vi "Get_Motor_Position.vi"(4 "Echo Mode (2)":i32=2, 6 "additional witing time (0)":u32, 7 "Motor In":u16(ring) items=["none", "1", "2", "3", "4", "all"], 8 "error in (no error)":errorcluster, 10 "Output Unit":T1=enum."Angle [TMC]", 11 "VISA resource name":refnum<visa-resource-name>) -> (0 "error out":errorcluster={"status"=FALSE, "code"=1073676294, "source"="VISA Read in write_read.vi"}, 1 "Position (Steps)":i32, 2 "Position":dbl, 3 "VISA ressource out":refnum<visa-resource-name>)   [LabVIEW 2018]
uses:
  ConversionAndInformation/Unit_Control.ctl
  MCode_LV_86/Set Parameter.ctl
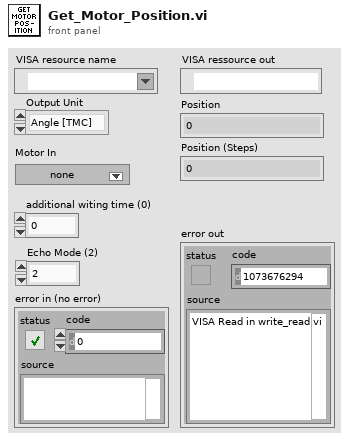
[diagram p1: front panel]
types:
  T1 = typedef "Unit_Control.ctl" = enum16{"Angle (Degrees)", "Rad", "Angle [TMC]", "Microsteps [TMC]", "Inches", "Nanometer", "Meter", "Centimeter", "Millimeter", "Micron"}
  T2 = typedef "Set Parameter.ctl" = enum16{"Acceleration (A)", "Baud Rate (BD)", "Counter 1 (C1)", "Counter 2 (C2)", "Control C Software Reset (CE)", "Check Sum Enable (CK)", "Clock Mode (CM)", "Clock Mode Ratio (CR)", "Clock Mode Out Step Width (CW)", "Deceleration (D)", "Digital Filtering, Input 1 (D1)", "Digital Filtering, Input 2 (D2)", "Digital Filtering, Input 3 (D3)", "Digital Filtering, Input 4 (D4)", "Digital Filtering, Input 5 (D5)", "Digital Filtering, Input 9 (D9)", "Digital Filtering, Input 10 (D10)", "Digital Filtering, Input 11 (D11)", "Digital Filtering, Input 12 (D12)", "Deadband (DB)", "Decrement Variable (DC)", "Enable/Disable Drive (DE)", "Device Name (DN)", "End Program Execution (E)", "Encoder Function Enable (EE)", "Error Flag (EF)", "Encoder Lines (EL)", "Echo Mode (EM)", "Error Value (ER)", "Escape (ES)", "Execute Program at Address (EX)", "Firmware Version (VR)", "Hold (H)", "Hold Current (HC)", "Hold Current Delay Time (HI)", "Home to Encoder Index (HM)", "Home to Home Switch (HT)", "Increment Variable (IC)", "Initialize Parameters to NVM (IP)", "Input into Variable (IV)", "Jog Enable (JE)", "Limit Stop Mode (LM)", "Move Absolute (MA)", "Move Relative (MR)", "MicroStepping Select (MS)", "Motor Settling Delay Time (MT)", "Moving [Flag] (MV)", "Output 1 (O1)", "Output 2 (O2)", "Output 3 (O3)", "Output 4 (O4)", "Output 9 (O9)", "Output 10 (O10)", "Output 11 (O11)", "Output 12 (O12)", "Output High Byte (9-12) (OH)", "Output Low Byte (1-4) (OL)", "Output Total (1-4 and 9-12) (OT)", "Position (P)", "Position Maintenance (PM)", "Party Mode (PY)", "Register 1 (R1)", "Register 2 (R2)", "Register 3 (R3)", "Register 4 (R4)", "Reset Error(\\03)", "Run Current (RC)", "Stall Factor (SF)", "Slew (SL)", "Stall Mode Set (SM)", "Upgrade Firmware (UG)", "Velocity Initial (VI)", "Velocity Maximum (VM)", "Current1 (I1)", "Current2 (I2)", "Current3 (I3)", "Current4 (I4)", "Current5 (I5)", "Current6 (I6)", "Save (S)"}
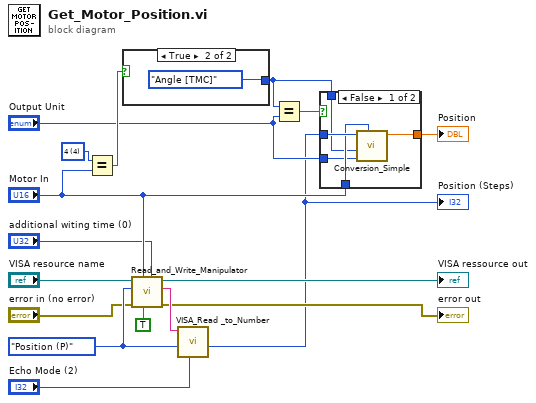
[diagram p0: block diagram]
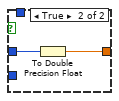
[diagram p2: hidden frame]
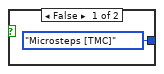
[diagram p3: hidden frame]
diagram:
  w9 = u16 4 items=["none", "1", "2", "3", "4", "all"] ("Motor")
  w15 = Set_Parameter."Position (P)" ("Command")
  n1 = Equal?(x=w9, y="Motor In") -> (x = y?=w7:bool)
  n2 = case shown="True" w7 {
    tunnel: [Unit_Control."Microsteps [TMC]" ("Input Unit") Unit_Control."Angle [TMC]" ("Input Unit")] -> w4
    frame False {
    }
    frame True {
    }
  }
  n3 = call "Read_and_Write_Manipulator.vi"("additional waiting time (0)"="additional witing time (0)", "Print?"=TRUE, "Motor"="Motor In", "error in (no error)"="error in (no error)", "Command"=w15, "VISA resource name"="VISA resource name") -> ("error out"=→"error out":errorcluster, "Answer"=w16:string, "VISA ressource out"=→"VISA ressource out":refnum<visa-resource-name>)  [unwired: 1 in, 2 out]
  n4 = call "VISA_Read _to_Number.vi"("Echo Mode"="Echo Mode (2)", "Command"=w15, "Answer Buffer"=w16) -> ("number (I32)"=w3:i32)  [unwired: 7 in, 1 out]
  "Position (Steps)" <- w3
  n5 = Equal?(x=w4, y="Output Unit") -> (x = y?=w6:bool)
  n6 = case shown="False" w6 {
    tunnel: w3 -> [w24 w26]
    tunnel: [w23 w25] -> w14
    tunnel: "Motor In" -> [w22 _]
    tunnel: w4 -> [w21 _]
    tunnel: "Output Unit" -> [w20 _]
    frame False {
      n7 = call "Conversion_Simple.vi"("Motor"=w22, "Output Unit"=w20, "Input Unit"=w21, "Input"=w24) -> ("Output"=w23:dbl)  [unwired: 6 in, 1 out]
    }
    frame True {
      n8 = To Double Precision Float(number=w26) -> (double precision float=w25:dbl)
    }
  }
  "Position" <- w14
